vi "CVT1StaticReadTest.vi"() -> (3 "Unit Test Framework Results":T1)   [LabVIEW 2013, in "UnitTests.lvlib"]
uses:
  UnitTests.lvlib
  <vilib>/utf/common/utf_test_result_troll.ctl
  <vilib>/utf/common/utf_test_result.ctl
  <vilib>/utf/common/utf_test_result_failure.ctl
  <vilib>/utf/common/utf_test_comparison_operators.ctl
  <vilib>/utf/common/utf_vi_tag.ctl
  <vilib>/NI/Current Value Table/Static Read.vi
  <vilib>/NI/Current Value Table/DataTypes/I32_Static Read.vi
  <vilib>/NI/Current Value Table/Type to Enum.vi
  <vilib>/NI/Current Value Table/DataTypes/I32_Type To Enum.vi
  <vilib>/NI/Current Value Table/Compatibility/TagConverter.vi
  <vilib>/NI/Current Value Table/Create Tags.vi
  <vilib>/NI/Current Value Table/FGVs/Tag Memory.vi
  <vilib>/NI/Current Value Table/Memory Block.vi
  <vilib>/NI/Current Value Table/DataTypes/I32_Memory Block.vi
  <vilib>/utf/NI_UnitTestFramework.lvlib
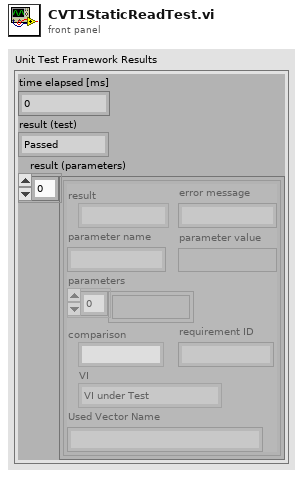
[diagram p1: front panel]
types:
  T1 = typedef "NI_UnitTestFramework.lvlib/utf_test_result_troll.ctl" = cluster{"time elapsed [ms]":u32, "result (test)":T2, "result (parameters)":T3[]}
  T2 = typedef "NI_UnitTestFramework.lvlib/utf_test_result.ctl" = enum16{"Passed", "Failed", "Error", "Skipped", "Not Processed"}
  T3 = typedef "NI_UnitTestFramework.lvlib/utf_test_result_failure.ctl" = cluster{"result":T2, "error message":string, "parameter name":string, "parameter value":variant, "parameters":variant[], "comparison":T4, "requirement ID":string, "VI":T5, "Used Vector Name":string}
  T4 = typedef "NI_UnitTestFramework.lvlib/utf_test_comparison_operators.ctl" = enum16{"=", "!=", ">", ">=", "<", "<=", "range", "symmetric tolerance", "asymmetric tolerance", "string contains", "string not contain", "array size", "string length", "array range", "by element", "array range (limit array)", "user-defined", "array contains", "array not contain", "vector length", "= (elm)", "!= (elm)", "= (case insensitive)", "!= (case insensitive)"}
  T5 = typedef "NI_UnitTestFramework.lvlib/utf_vi_tag.ctl" = enum16{"Setup VI", "VI under Test", "Teardown VI"}
  T6 = typedef "cvt_Tag Configuration.ctl" = cluster{"Name":string, "Data Type":T7, "Array":bool, "Size":u32, "Default":string, "Enum":string[], "Description":string}
  T7 = typedef "cvt_Data Types.ctl" = enum16{"Bool", "U8", "I32", "Double", "String", "Enum"}
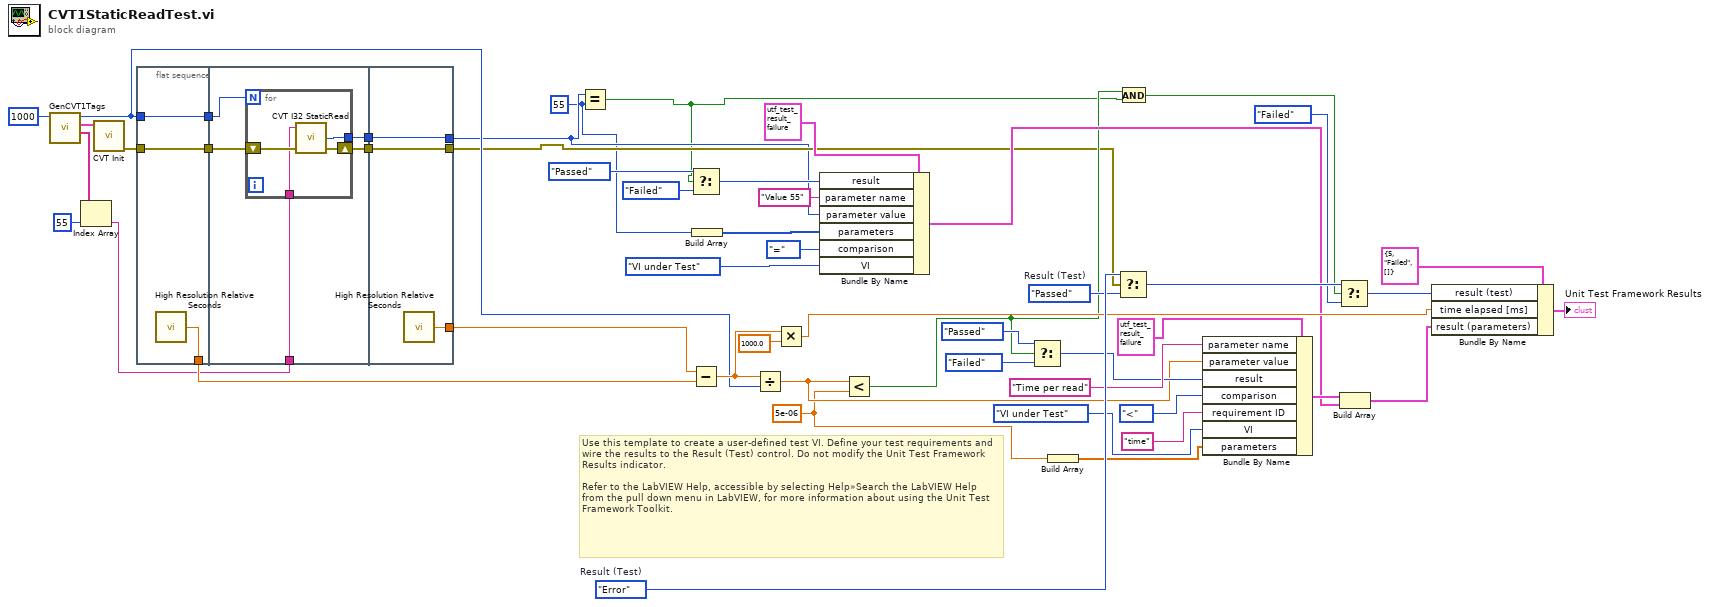
[diagram p0: block diagram]
diagram:
  w5 = 55 ("y")
  w21 = 5e-06 ("y")
  w46 = utf_test_result."Error"  # Result (Test)
  w45 = utf_test_result."Passed"  # Result (Test)
  # "Use this template to create a user-defined test VI. Define your test requirements and wire the results to the Result (Test) control. Do not modify the Unit Test Framework Results indicator. \n\nRefer to the LabVIEW Help, accessible by selecting Help»Search the LabVIEW Help from the pull down menu in LabVIEW, for more information about using the Unit Test Framework Toolkit."
  n1 = call "GenCVT1Tags.vi"("Number of Tags in"=1000) -> ("Names"=w3:string[], "Tags"=w39:T6[], "Number of Tags out"=w32:i32)  [unwired: 8 in]
  n2 = Index Array(array=w3, index=55) -> (element=w1:string)
  n3 = call <vilib>:"CVT Init.vi"("Tag List"=w39) -> ("error out"=w38:errorcluster)  [unwired: 10 in]
  n4 = flat-sequence {
    tunnel: [w54] -> w48
    tunnel: w38 -> [w52]
    tunnel: [w53] -> w37
    tunnel: w32 -> [w53]
    tunnel: [w52] -> w36
    tunnel: w37 -> [w59]
    tunnel: w36 -> [w58]
    tunnel: [w57] -> w35
    tunnel: [w56] -> w16
    tunnel: w1 -> [w55]
    tunnel: [w66] -> w49
    tunnel: w35 -> [w65]
    tunnel: [w65] -> w8
    tunnel: [w64] -> w7
    tunnel: w16 -> [w64]
    frame #0 {
      n5 = call <vilib>:"High Resolution Relative Seconds.vi"() -> ("relative seconds"=w54:dbl)
    }
    frame #1 {
      n6 = for {
        N: w59 -> [_]
        shift-right: [w62] -> w57
        shift-left: w58 -> [w63]
        tunnel: [w61] -> w56
        tunnel: w55 -> [w60]
        n7 = call <vilib>:"CVT I32 StaticRead.vi"("error in (no error)"=w63, "Tag Name"=w60) -> ("error out"=w62:errorcluster, "Value"=w61:i32)  [unwired: 2 in]
      }
    }
    frame #2 {
      n8 = call <vilib>:"High Resolution Relative Seconds.vi"() -> ("relative seconds"=w66:dbl)
    }
  }
  n9 = Equal?(x=w7, y=w5) -> (x = y?=w6:bool)
  n10 = Select(t=utf_test_result."Passed" ("result"), s=w6, f=utf_test_result."Failed" ("result")) -> (s? t:f=w11:T2)
  n11 = Subtract(x=w49, y=w48) -> (x-y=w34:dbl)
  n12 = Build Array(w5) -> (w9:i32[])
  n13 = Divide(x=w34, y=w32) -> (x/y=w24:dbl)
  n14 = Multiply(x=w34, y=1000.0) -> (x*y=w40:dbl)
  n15 = Bundle By Name(cluster=T3 {"result"=enum."Passed", "error message"="", "parameter name"="", "parameter value"=variant, "parameters"=[], "comparison"=enum."=", "requirement ID"="", "VI"=enum."Setup VI", "Used Vector Name"=""} ("Unit Test Framework - result (parameters)"), "result"=w11, "parameter name"="Value 55", "parameter value"=w7, "parameters"=w9, "comparison"=utf_test_comparison_operators."=", "VI"=utf_vi_tag."VI under Test") -> (w19:T3)
  n16 = Less?(x=w24, y=w21) -> (x < y?=w17:bool)
  n17 = Select(t=utf_test_result."Passed" ("result"), s=w17, f=utf_test_result."Failed" ("result")) -> (s? t:f=w25:T2)
  n18 = Build Array(w21) -> (w20:dbl[])
  n19 = Select(t=w46, s=w8, f=w45) -> (s? t:f=w31:T2)
  n20 = And(x=w17, y=w6) -> (x .and. y?=w18:bool)
  n21 = Bundle By Name(cluster=T3 {"result"=enum."Passed", "error message"="", "parameter name"="", "parameter value"=variant, "parameters"=[], "comparison"=enum."=", "requirement ID"="", "VI"=enum."Setup VI", "Used Vector Name"=""} ("Unit Test Framework - result (parameters)"), "parameter name"="Time per read", "parameter value"=w24, "result"=w25, "comparison"=utf_test_comparison_operators."<", "requirement ID"="time", "VI"=utf_vi_tag."VI under Test", "parameters"=w20) -> (w43:T3)
  n22 = Select(t=w31, s=w18, f=utf_test_result."Failed") -> (s? t:f=w29:T2)
  n23 = Build Array(w43, w19) -> (w42:T3[])
  n24 = Bundle By Name(cluster=T1 {"time elapsed [ms]"=5, "result (test)"=enum."Failed", "result (parameters)"=[]} ("Unit Test Framework - Result"), "result (test)"=w29, "time elapsed [ms]"=w40, "result (parameters)"=w42) -> (→"Unit Test Framework Results":T1)
